vi "redukuj wektor.vi"(6 "length (320)":i32=320, 7 "redukuj":bool=TRUE, 11 "Waveform in":waveform(dbl)) -> (3 "Waveform out":waveform(dbl))   [LabVIEW 2014]
doc: "redukuje długość wektora (początkowa 390)\ndługość 320 - 0,1s\ndługość 384 - 0,12s"
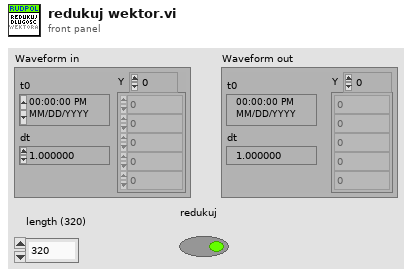
[diagram p1: front panel]
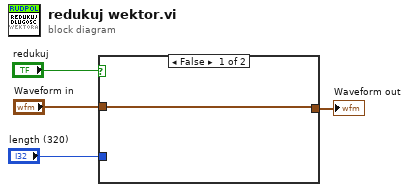
[diagram p0: block diagram]
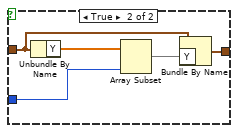
[diagram p2: hidden frame]
diagram:
  n1 = case shown="False" "redukuj" {
    tunnel: [w5 w10] -> w4
    tunnel: "Waveform in" -> [w5 w9]
    tunnel: "length (320)" -> [_ w7]
    frame False {
    }
    frame True {
      n2 = Unbundle By Name(w9) -> ("Y"=w6:dbl[])
      n3 = Array Subset(array=w6, length=w7) -> (w8:dbl[])  [unwired: 1 in]
      n4 = Bundle By Name(cluster=w9, "Y"=w8) -> (w10:waveform(dbl))
    }
  }
  "Waveform out" <- w4
